vi "call dll with path.vi"() -> ()   [LabVIEW 2020]
uses:
  GPS_SIM_CREATE_BIN_32.dll
panel:
  out "deleted path":path
  in  "text":string
  out "dll exit":bool
  out "error out 2":errorcluster
  in  "stop":bool
  out "base_path":string="C:\\Users\\duyga\\OneDrive\\??????\\WORKS\\Nissan GPS\\gps-sdr-sim-dll - add base path"
  out "error out":errorcluster
  in  "param":string="-e brdc0010.22n -u circle.csv -d 10 -o filename"
  out "return code":i32
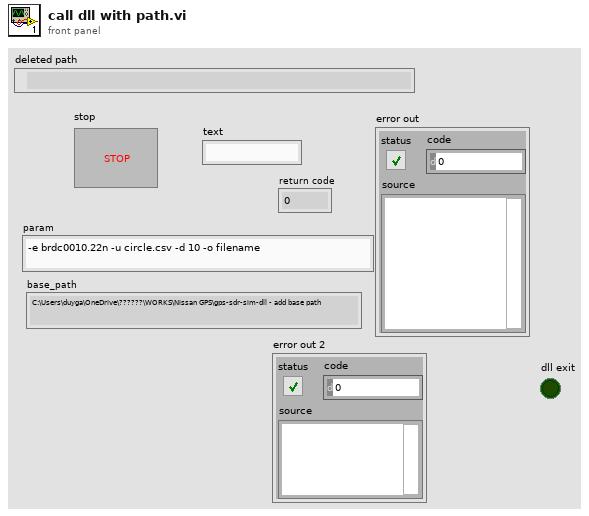
[diagram p1: front panel]
types:
  T1 = enum16{"open", "replace", "create", "open or create", "replace or create", "replace or create with confirmation"}
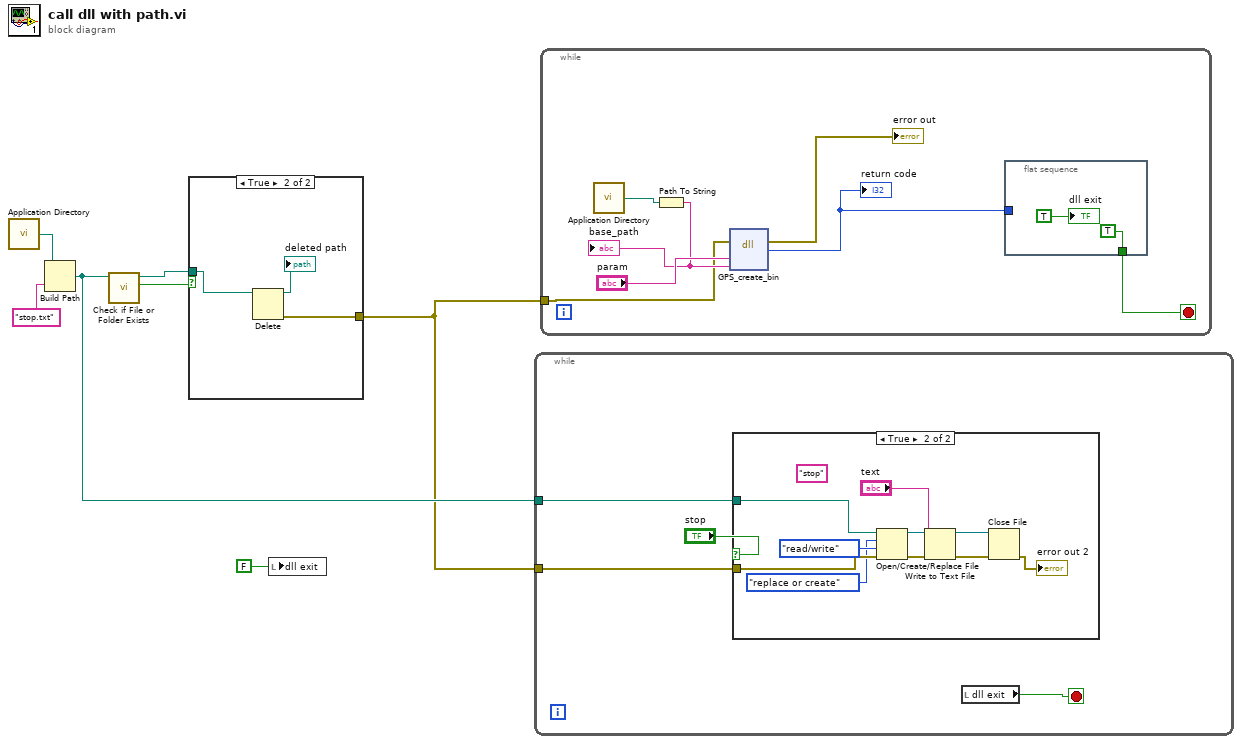
[diagram p0: block diagram]
diagram:
  n1 = call <vilib>:"Application Directory.vi"() -> ("Application Directory"=w7:path)
  n2 = Build Path(base path=w7, name or relative path="stop.txt") -> (appended path=w4:path)
  n3 = call <vilib>:"Check if File or Folder Exists.vi"("path"=w4) -> ("file or folder exists?"=w3:bool, "dup path"=w2:path)  [unwired: 8 in, 1 out]
  n4 = case shown="True" w3 {
    tunnel: w2 -> [_ w10]
    tunnel: [_ w9] -> w1
    frame False {
    }
    frame True {
      n5 = Delete(path (use dialog)=w10) -> (deleted path=→"deleted path":path, error out=w9:errorcluster)  [unwired: 4 in, 1 out]
    }
  }
  n6 = local write "dll exit"(FALSE ("dll exit")) -> ()
  n7 = while {
    tunnel: w1 -> [w14]
    tunnel: w4 -> [w13]
    stop <- w12 stop-if-true
    n8 = case shown="True" "stop" {
      tunnel: w13 -> [_ w20]
      tunnel: w14 -> [_ w19]
      frame False {
      }
      frame True {
        (unwired) "stop" ("text")
        n9 = Open/Create/Replace File(file path (use dialog)=w20, error in=w19, operation (0:open)=T1."replace or create", access (0:read/write)=enum16{"read/write", "read-only", "write-only"}."read/write") -> (refnum out=w15:refnum<file>, error out=w18:errorcluster)  [unwired: 2 in, 1 out]
        n10 = Write to Text File(file (use dialog)=w15, text="text", error in=w18) -> (refnum out=w21:refnum<file>, error out=w22:errorcluster)  [unwired: 1 in, 1 out]
        n11 = Close File(refnum=w21, error in=w22) -> (error out=→"error out 2":errorcluster)  [unwired: 1 out]
      }
    }
    n12 = local read "dll exit"() -> (w12:bool)
  }
  n13 = while {
    tunnel: w1 -> [w25]
    stop <- w26 stop-if-true
    n14 = call <vilib>:"Application Directory.vi"() -> ("Application Directory"=w29:path)
    n15 = Path To String(path=w29) -> (string=w28:string)
    "base_path" <- w28
    n16 = dll-call lib="PTH2labs CUsersduygaOneDriveデスクトップWORKS\nNissan GPS\tbuild dllGPS_SIM_CREATE_BIN_32.dll" fn="GPS_create_bin"(error in=w25, "param"="param", "base_path"=w28) -> (error out=→"error out":errorcluster, "return code"=w27:i32)  [unwired: 4 in, 1 out]
    "return code" <- w27
    n17 = flat-sequence {
      tunnel: w27 -> [_]
      tunnel: [TRUE] -> w26
      frame #0 {
        "dll exit" <- TRUE ("dll exit")
      }
    }
  }
